vi "LaserCal-Set Icon Color.vi"(7 "Color":u32(colorbox)) -> (8 "2D Picture":picture)   [LabVIEW 2015]
uses:
  <vilib>/picture/picture.llb/Draw True-Color Pixmap.vi
panel:
  out "min value":u8
  out "max value":u8
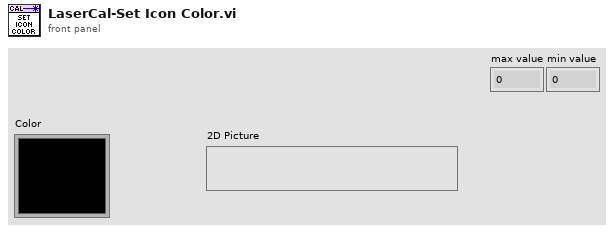
[diagram p1: front panel]
types:
  T1 = typedef "imagedata.ctl" = cluster{"image type":i32, "image depth":i32, "image":u8[], "mask":u8[], "colors":u32[], "Rectangle":cluster{"left":i16, "top":i16, "right":i16, "bottom":i16}}
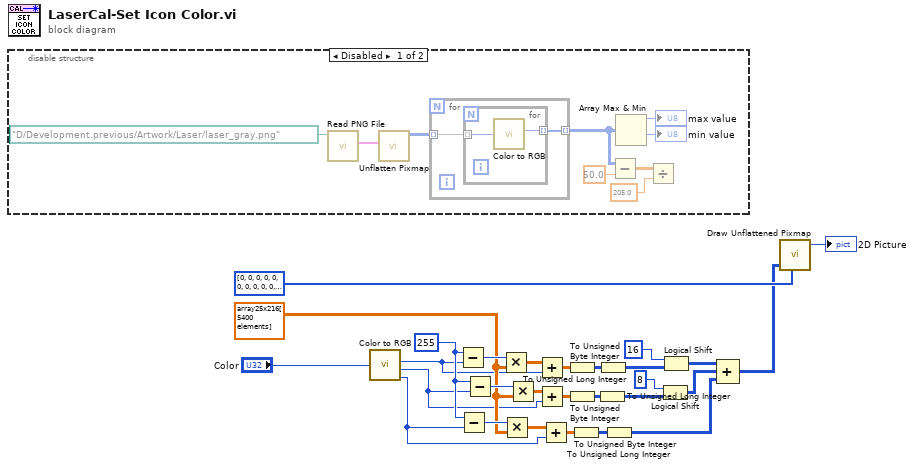
[diagram p0: block diagram]
diagram:
  w7 = dbl[][] array25x216[5400 elements] ("x/y")
  w9 = u8 255 ("x")
  n1 = disable-structure shown="Disabled" {
    frame Disabled {
      n2 = call <vilib>:"Read PNG File.vi"("path to PNG file"=path "D:/Development.previous/Artwork/Laser/laser_gray.png") -> ("image data"=w36:T1)  [unwired: 8 in, 2 out]
      n3 = call <vilib>:"Unflatten Pixmap.vi"("image data"=w36) -> ("24-bit pixmap"=w35:u32[][])  [unwired: 4 in, 6 out]
      n4 = for {
        tunnel: w35 -> [w39] mode=indexing
        tunnel: [w38] -> w32 mode=indexing
        n5 = for {
          tunnel: w39 -> [w41] mode=indexing
          tunnel: [w40] -> w38 mode=indexing
          n6 = call <vilib>:"Color to RGB.vi"("Color"=w41) -> ("R"=w40:u8)  [unwired: 3 out]
        }
      }
      n7 = Subtract(x=w32, y=50.0) -> (x-y=w30:dbl[][])
      n8 = Array Max & Min(array=w32) -> (max value=→"max value":u8, min value=→"min value":u8)  [unwired: 2 out]
      n9 = Divide(x=w30, y=205.0) -> ()  [unwired: 1 out]
    }
    frame Enabled {
    }
  }
  n10 = call <vilib>:"Color to RGB.vi"("Color"="Color") -> ("R"=w2:u8, "G"=w4:u8, "B"=w3:u8)  [unwired: 1 out]
  n11 = Subtract(x=w9, y=w2) -> (x-y=w14:u8)
  n12 = Subtract(x=w9, y=w3) -> (x-y=w10:u8)
  n13 = Subtract(x=w9, y=w4) -> (x-y=w12:u8)
  n14 = Multiply(x=w14, y=w7) -> (x*y=w13:dbl[][])
  n15 = Multiply(x=w10, y=w7) -> (x*y=w5:dbl[][])
  n16 = Multiply(x=w12, y=w7) -> (x*y=w11:dbl[][])
  n17 = Add(x=w13, y=w2) -> (x+y=w27:dbl[][])
  n18 = Add(x=w11, y=w4) -> (x+y=w25:dbl[][])
  n19 = Add(x=w5, y=w3) -> (x+y=w24:dbl[][])
  n20 = To Unsigned Byte Integer(number=w27) -> (unsigned 8bit integer=w23:u8[][])
  n21 = To Unsigned Byte Integer(number=w25) -> (unsigned 8bit integer=w19:u8[][])
  n22 = To Unsigned Byte Integer(number=w24) -> (unsigned 8bit integer=w18:u8[][])
  n23 = To Unsigned Long Integer(number=w19) -> (unsigned 32bit integer=w6:u32[][])
  n24 = To Unsigned Long Integer(number=w23) -> (unsigned 32bit integer=w21:u32[][])
  n25 = To Unsigned Long Integer(number=w18) -> (unsigned 32bit integer=w15:u32[][])
  n26 = Logical Shift(y=i16 8, x=w6) -> (x << y=w16:u32[][])
  n27 = Logical Shift(y=i16 16, x=w21) -> (x << y=w17:u32[][])
  n28 = Compound Arithmetic op=ADD(w17, w16, w15) -> (w8:u32[][])
  n29 = call-poly <vilib>:"Draw Unflattened Pixmap.vi"("data (RGB format)"=w8, "mask"=u8[] [0, 0, 0, 0, 0, 0, 0, 0, 0, 0, 0, 0, 0, 0, 0, 0, 0, 0, 0, 0, 0, 0, 0, 0, 0, 64, 0, 0, 0, 0, 0, 0, 0, 0, 0, 0, 0, 0, 0, 0, 0, 0, 0, 0, 0, 0, 0, 0, 0, 0, 0, 0, 0, 96, 0, 0, 0, 0, 0, 0, 0, 0, 0, 0, 0, 0, 0, 0, 0, 0, 0, 0, 0, 0, 0, 0, 0, 0, 0, 0, 0, 32, 0, 0, 0, 0, 0, 0, 0, 0, 0, 0, 0, 0, 0, 0, 0, 0, 0, 0, 0, 0, 0, 0, 0, 0, 0, 0, 0, 49, 0, 0, 0, 0, 0, 0, 0, 0, 0, 0, 0, 0, 0, 0, 0, 0, 0, 0, 0, 0, 0, 0, 0, 0, 0, 0, 0, 57, 128, 0, 0, 0, 0, 0, 0, 0, 0, 0, 0, 0, 0, 0, 0, 0, 0, 0, 0, 0, 0, 0, 0, 0, 0, 0, 1, 29, 128, 0, 0, 0, 0, 0, 0, 0, 0, 0, 0, 0, 0, 0, 0, 0, 0, 0, 0, 0, 0, 0, 0, 0, 0, 0, 1, 223, 208, 0, 0, 0, 0, 0, 0, 0, 0, 0, 0, 0, 0, 0, 0, 0, 0, 0, 0, 0, 0, 0, 0, 0, 0, 0, 1, 255, 240, 0, 0, 0, 0, 0, 0, 0, 0, 0, 0, 0, 0, 0, 0, 0, 0, 0, 0, 0, 0, 0, 0, 0, 0, 0, 0, 255, 224, 0, 0, 0, 0, 0, 0, 0, 0, 0, 0, 0, 0, 0, 0, 0, 0, 0, 0, 0, 0, 0, 0, 0, 0, 0, 0, 127, 240, 0, 255, 255, 255, 255, 255, 255, 255, 255, 255, 255, 255, 255, 255, 255, 255, 255, 255, 255, 255, 255, 255, 255, 255, 255, 255, 255, 252, 0, 255, 255, 255, 255, 255, 255, 255, 255, 255, 255, 255, 255, 255, 255, 255, 255, 255, 255, 255, 255, 255, 255, 255, 255, 255, 255, 255, 0, 255, 255, 255, 255, 255, 255, 255, 255, 255, 255, 255, 255, 255, 255, 255, 255, 255, 255, 255, 255, 255, 255, 255, 255, 255, 255, 252, 0, 255, 255, 255, 255, 255, 255, 255, 255, 255, 255, 255, 255, 255, 255, 255, 255, 255, 255, 255, 255, 255, 255, 255, 255, 255, 255, 240, 0, 255, 255, 255, 255, 255, 255, 255, 255, 255, 255, 255, 255, 255, 255, 255, 255, 255, 255, 255, 255, 255, 255, 255, 255, 255, 255, 240, 0, 0, 0, 0, 0, 0, 0, 0, 0, 0, 0, 0, 0, 0, 0, 0, 0, 0, 0, 0, 0, 0, 0, 0, 0, 0, 255, 248, 0, 0, 0, 0, 0, 0, 0, 0, 0, 0, 0, 0, 0, 0, 0, 0, 0, 0, 0, 0, 0, 0, 0, 0, 0, 1, 255, 248, 0, 0, 0, 0, 0, 0, 0, 0, 0, 0, 0, 0, 0, 0, 0, 0, 0, 0, 0, 0, 0, 0, 0, 0, 0, 3, 255, 252, 0, 0, 0, 0, 0, 0, 0, 0, 0, 0, 0, 0, 0, 0, 0, 0, 0, 0, 0, 0, 0, 0, 0, 0, 0, 7, 255, 128, 0, 0, 0, 0, 0, 0, 0, 0, 0, 0, 0, 0, 0, 0, 0, 0, 0, 0, 0, 0, 0, 0, 0, 0, 0, 6, 63, 192, 0, 0, 0, 0, 0, 0, 0, 0, 0, 0, 0, 0, 0, 0, 0, 0, 0, 0, 0, 0, 0, 0, 0, 0, 0, 0, 63, 128, 0, 0, 0, 0, 0, 0, 0, 0, 0, 0, 0, 0, 0, 0, 0, 0, 0, 0, 0, 0, 0, 0, 0, 0, 0, 0, 115, 128, 0, 0, 0, 0, 0, 0, 0, 0, 0, 0, 0, 0, 0, 0, 0, 0, 0, 0, 0, 0, 0, 0, 0, 0, 0, 0, 97, 128, 0, 0, 0, 0, 0, 0, 0, 0, 0, 0, 0, 0, 0, 0, 0, 0, 0, 0, 0, 0, 0, 0, 0, 0, 0, 0, 65, 128, 0, 0, 0, 0, 0, 0, 0, 0, 0, 0, 0, 0, 0, 0, 0, 0, 0, 0, 0, 0, 0, 0, 0, 0, 0, 0, 0, 0, 0]) -> ("new picture"=→"2D Picture":picture)  [unwired: 7 in]
